vi "Read airmass.vi"(8 "error in (no error)":errorcluster, 11 "AmLimit in":refnum<class "AmLimit.lvclass">) -> (0 "error out":errorcluster, 2 "airmass":dbl=3.0 min=1.0 max=15.0, 3 "AmLimit out":refnum<class "AmLimit.lvclass">)   [LabVIEW 2022 SP3, in "TCSDataDefinitions.lvlib" / "TCSCommand.lvlib" / "AmLimit.lvclass"]
uses:
  AmLimit.lvclass
  AmLimit.lvclass/AmLimit.ctl
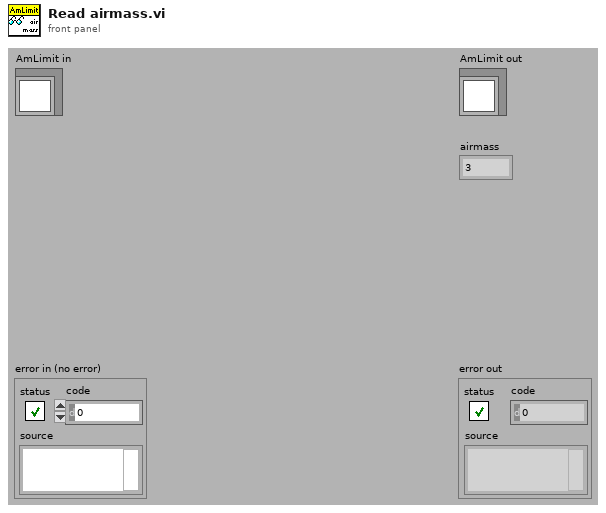
[diagram p1: front panel]
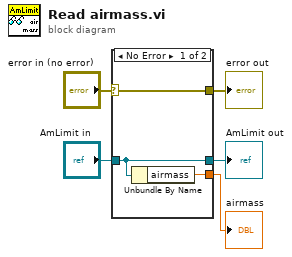
[diagram p0: block diagram]
diagram:
  n1 = case shown="No Error" "error in (no error)" {
    selector: "error in (no error)" -> [w8 w9]
    tunnel: [w8 w9] -> w4
    tunnel: [w7 w10] -> w2
    tunnel: "AmLimit in" -> [w7 w10]
    tunnel: [w6 _] -> w1
    frame No Error {
      n2 = Unbundle By Name(w7) -> ("airmass"=w6:dbl)
    }
    frame Error {
    }
  }
  "error out" <- w4
  "AmLimit out" <- w2
  "airmass" <- w1
